vi "Experiment_1.vi"() -> ()   [LabVIEW 2019]
uses:
  <vilib>/measure/NI_MABase.lvlib
panel:
  in  "signal type":T1(ring)
  in  "phase":dbl format="%.2p"
  out "Demodulated Signal":dynamicdata(graph)=[{"t0"=timestamp(0 s since 1904-01-01), "dt"=0.0001, "Y"=array[1000 elements], "attributes"=variant("NI_ChannelName"=variant(string "Filtered"))}]
  out "Modulated Signal":waveform(dbl)(graph)={"t0"=timestamp(0 s since 1904-01-01), "dt"=0.0001, "Y"=array[1000 elements]}
  out "Carrier Signal":waveform(dbl)(graph)={"t0"=timestamp(0 s since 1904-01-01), "dt"=0.0001, "Y"=array[1000 elements]}
  out "Modulating Signal":waveform(dbl)(graph)={"t0"=timestamp(0 s since 1904-01-01), "dt"=0.0001, "Y"=array[1000 elements]}
  in  "amplitude 2":dbl=1.0 format="%0.2p"
  in  "frequency 2":dbl=1000.0 format="%0.2p"
  in  "sampling info":cluster{"Fs":dbl, "#s":dbl}={"Fs"=10000.0, "#s"=1000.0} {"Fs" format="%.2p"}
  in  "amplitude":dbl=1.0 format="%0.2p"
  in  "frequency":dbl=10.0 format="%0.2p"
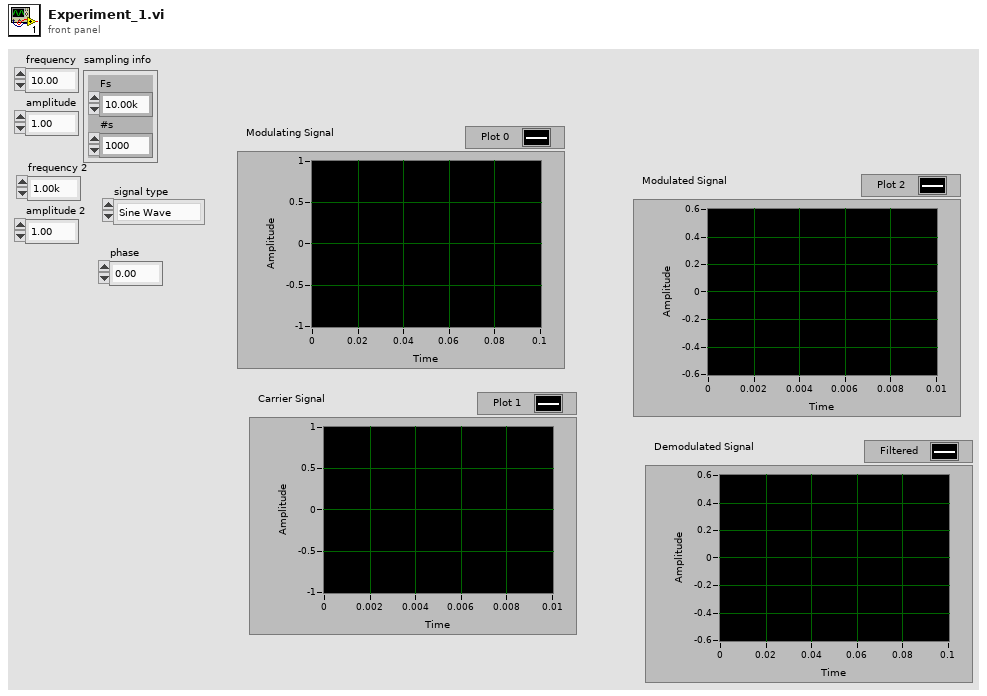
[diagram p1: front panel]
types:
  T1 = enum16{"Sine Wave", "Triangle Wave", "Square Wave", "Sawtooth Wave"}
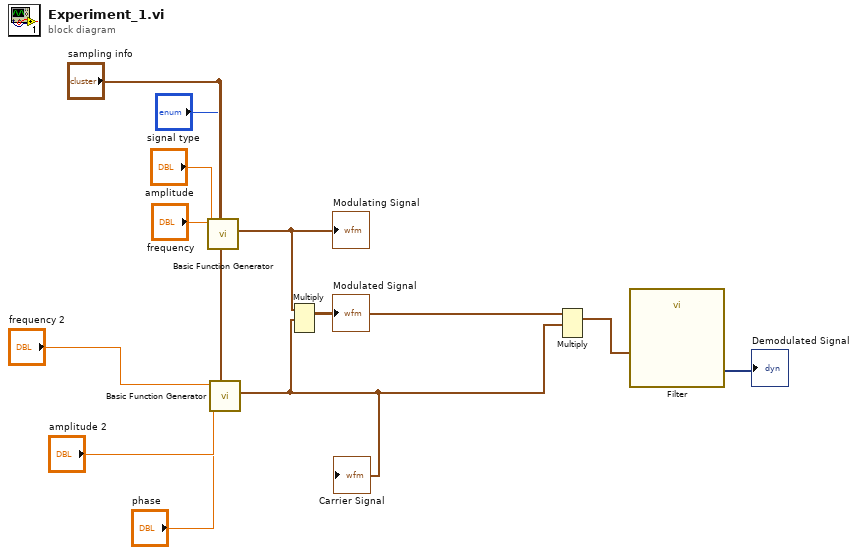
[diagram p0: block diagram]
diagram:
  n1 = call <vilib>:"Basic Function Generator.vi"("sampling info"="sampling info", "signal type"="signal type", "amplitude"="amplitude", "frequency"="frequency") -> ("signal out"=w7:waveform(dbl))  [unwired: 5 in, 2 out]
  "Modulating Signal" <- w7
  n2 = call <vilib>:"Basic Function Generator.vi"("sampling info"="sampling info", "phase"="phase", "amplitude"="amplitude 2", "frequency"="frequency 2") -> ("signal out"=w5:waveform(dbl))  [unwired: 5 in, 2 out]
  "Carrier Signal" <- w5
  n3 = Multiply(1:w5, 2:w7) -> (0:w6:waveform(dbl))  [unwired: 1 in, 1 out]
  "Modulated Signal" <- w6
  n4 = Multiply(1:w5, 2:w6) -> (0:w4:waveform(dbl))  [unwired: 1 in, 1 out]
  n5 = call "Filter"("Signal"=w4) -> ("Filtered Signal"=→"Demodulated Signal":dynamicdata)  [unwired: 9 in, 1 out]
